vi "ReadJSONFromSerialPort.vi"() -> ()   [LabVIEW 2022 SP3]
uses:
  <vilib>/Analysis/coordinate.llb/Angle Range (Degree).ctl
  <vilib>/Analysis/coordinate.llb/Angle Units.ctl
  <vilib>/Analysis/coordinate.llb/Wrap Angle (scalar).vi
  <vilib>/Instr/_visa.llb/VISA Configure Serial Port (Instr).vi
  <vilib>/addons/control/pid/pid.llb/PID Advanced (DBL).vi
  <vilib>/addons/control/pid/NI_PID_pid.lvlib
  <vilib>/Analysis/NI_AAL_Angle.lvlib
panel:
  in  "auto? (T)":bool=TRUE
  in  "manual output":dbl format="%.2f"
  out "Arduino meas speed RPM":dbl(graph)
  out "LabviewRPM":dbl(graph)
  out "rpm":dbl
  out "angle":dbl(knob) scale=0.0..360.0
  out "force":dbl(graph)
  out "Speed Indicator":dbl=20.0
  in  "Tf [s]":dbl=5.0 caption="Filter time-constant, Tf [s]" min=0.0
  out "PID out":dbl(graph)
  in  "PID gains":T1={"proportional gain (Kc)"=1.0, "integral time (Ti, min)"=0.01, "derivative time (Td, min)"=0.0} {"derivative time (Td, min)" format="%.3f"; "integral time (Ti, min)" format="%.3f"; "proportional gain (Kc)" format="%.3f"}
  in  "setpoint":dbl format="%.2f"
  out "error out 3":errorcluster
  out "measured loop time":dbl
  out "Json out":string
  out "speed chart":T2(graph)
  out "angleChart":dbl(graph)
  in  "stop":bool
  out "angle 2":dbl
  out "error out":errorcluster
  out "Json in":string
  in  "baud rate (115200)":u32=250000
  in  "VISA resource name 2":refnum<visa-resource-name>="COM3"
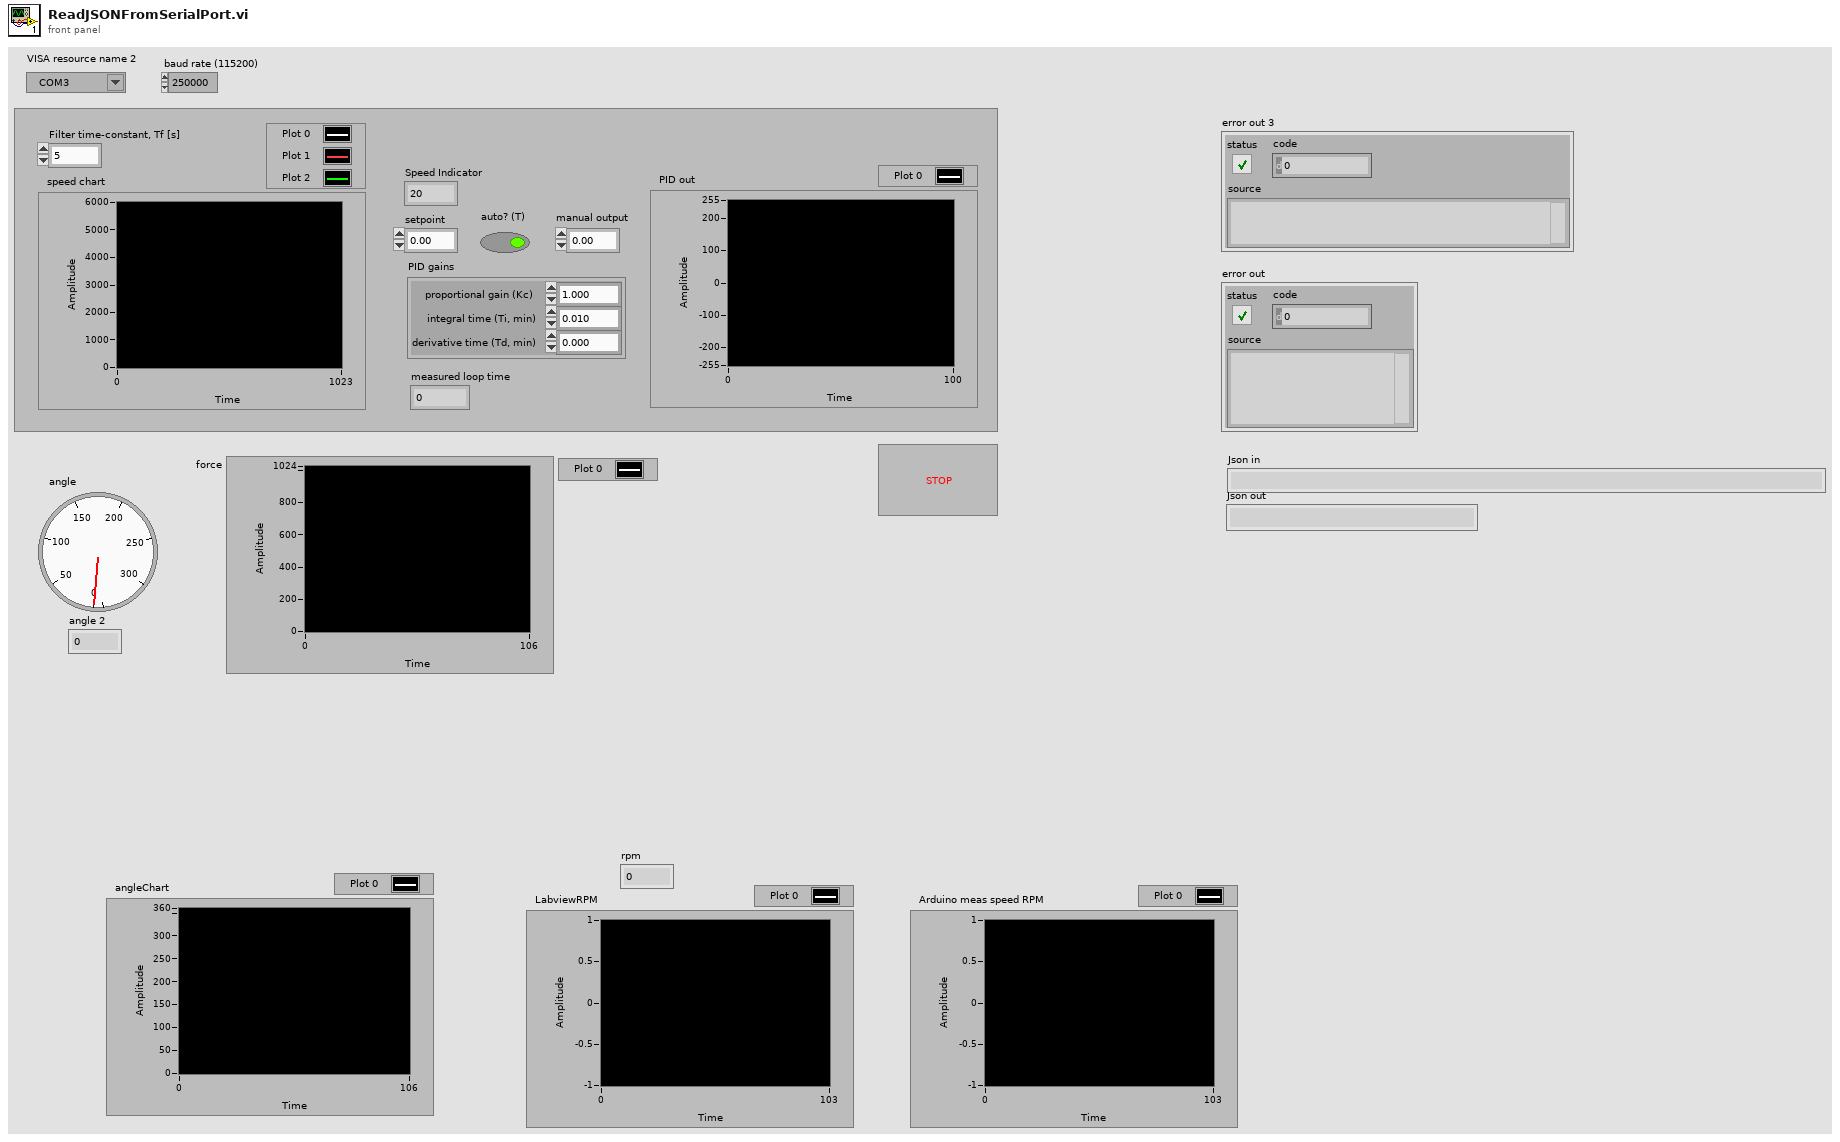
[diagram p1: front panel]
types:
  T1 = cluster{"proportional gain (Kc)":dbl, "integral time (Ti, min)":dbl, "derivative time (Td, min)":dbl}
  T2 = cluster{"setpoint":dbl, "Filter_output":dbl, "speed":dbl}
  T3 = typedef "NI_AAL_Angle.lvlib/Angle Units.ctl" = i32
  T4 = typedef "NI_AAL_Angle.lvlib/Angle Range (Degree).ctl" = u16
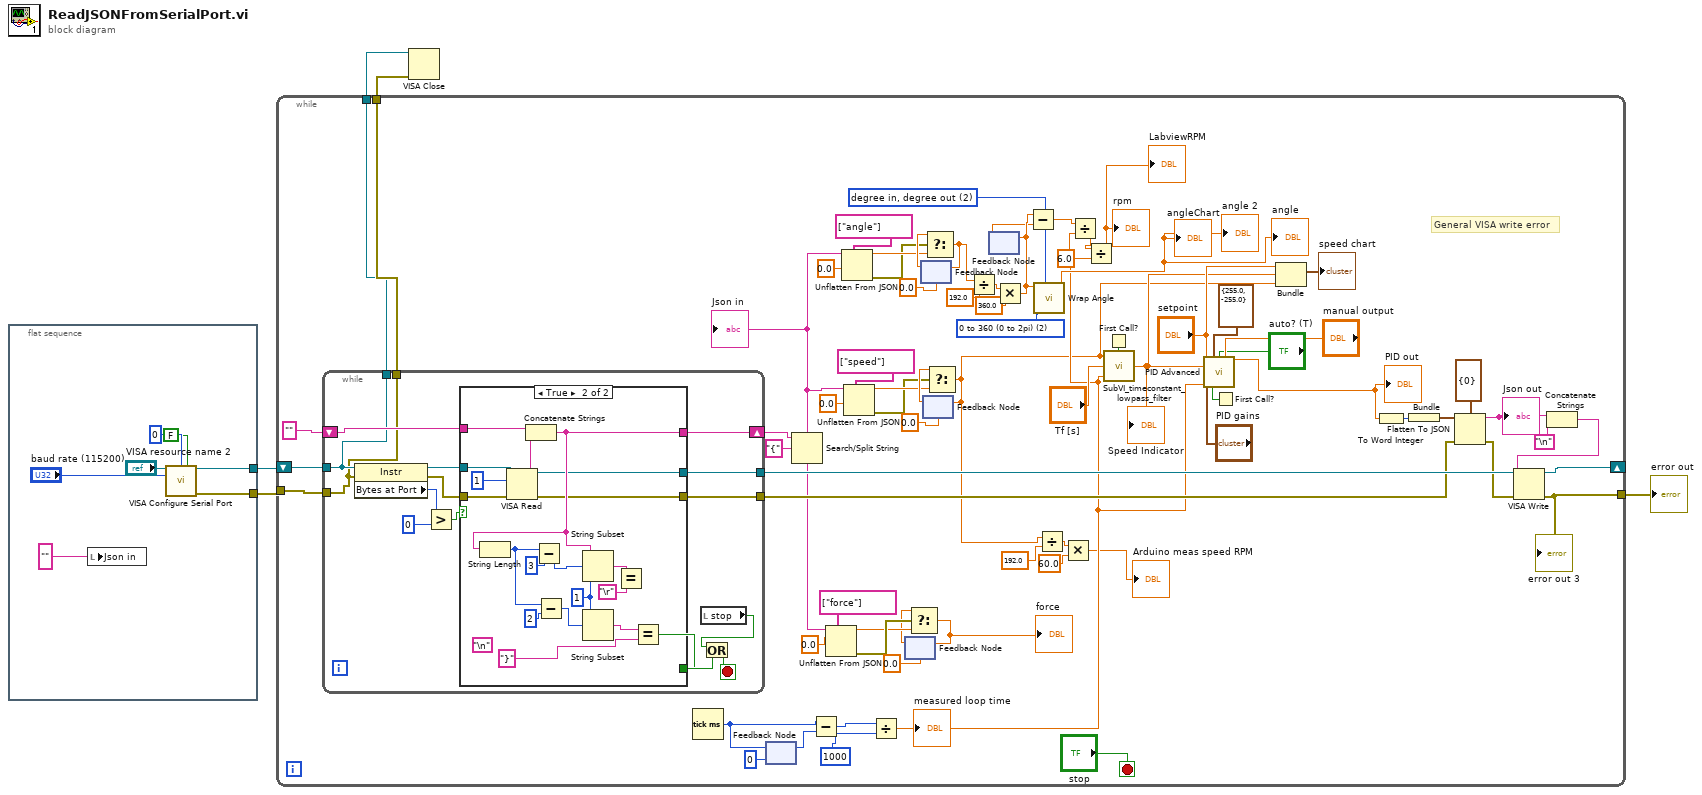
[diagram p0: block diagram]
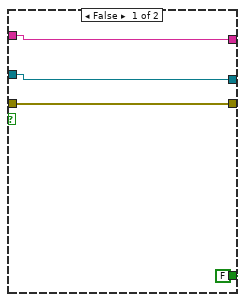
[diagram p2: hidden frame]
diagram:
  n1 = flat-sequence {
    tunnel: [w10] -> w1
    tunnel: [w9] -> w5
    frame #0 {
      n2 = local write "Json in"("" ("data string")) -> ()
      n3 = call-poly "VISA Configure Serial Port"("VISA resource name"="VISA resource name 2", "termination char\n(0xA = '\\n' = LF)"=u8 0 ("termination char\n(0xA = '\\n' = LF)"), "Enable Termination\nChar (T)"=FALSE ("Enable Termination\nChar (T)"), "baud rate (9600)"="baud rate (115200)") -> ("VISA resource name out"=w10:refnum<visa-resource-name>, "error out"=w9:errorcluster)  [unwired: 10 in]
    }
  }
  n4 = while {
    tunnel: w5 -> [w86]
    tunnel: [w84] -> w4
    tunnel: [w83] -> w3
    tunnel: [w71] -> w2
    shift-right: [w67] -> _
    shift-left: w1 -> [w66]
    stop <- "stop" stop-if-true
    w32 = T3 2 items=["radian in, radian out", "radian in, degree out", "degree in, degree out", "degree in, radian out"] ("angle units")
    w33 = T4 2 items=["none", "-180 to 180 (-pi to pi)", "0 to 360 (0 to 2pi)"] ("angle range")
    # "General VISA write error"
    n5 = while {
      tunnel: w66 -> [w93]
      tunnel: w86 -> [w92]
      shift-right: [w95] -> w54
      shift-left: "" -> [w94]
      tunnel: [w93] -> w83
      tunnel: [w92] -> w84
      tunnel: [w91] -> w47
      tunnel: [w87] -> w72
      stop <- w89 stop-if-true
      n6 = property class="Instr"(reference=w93, error in=w92) -> (reference out=w99:refnum<visa-resource-name>, error out=w100:errorcluster, "Bytes at Port"=w98:u32)
      n7 = Greater?(x=w98, y=u32 0) -> (0:w96:bool)
      n8 = case shown="True" w96 {
        tunnel: w100 -> [w102 w123]
        tunnel: w99 -> [w101 w122]
        tunnel: [w104 w112] -> w95
        tunnel: w94 -> [w104 w119]
        tunnel: [FALSE w106] -> w90
        tunnel: [w102 w108] -> w91
        tunnel: [w101 w105] -> w87
        frame False {
        }
        frame True {
          (unwired) "\n"
          w114 = 1 ("length (rest)")
          n9 = VISA Read(VISA resource name=w122, byte count=u32 1, error in (no error)=w123) -> (VISA resource name out=w105:refnum<visa-resource-name>, read buffer=w120:string, error out=w108:errorcluster)  [unwired: 1 out]
          n10 = Concatenate Strings "Concatenate Strings"(w119, w120) -> (w112:string)
          n11 = String Length(string=w112) -> (length=w117:i32)
          n12 = Subtract(x=w117, y=3) -> (x-y=w115:i32)
          n13 = Subtract(x=w117, y=2) -> (x-y=w113:i32)
          n14 = String Subset(string=w112, offset (0)=w115, length (rest)=w114) -> (substring=w111:string)
          n15 = String Subset(string=w112, offset (0)=w113, length (rest)=w114) -> (substring=w109:string)
          n16 = Equal?(x=w111, y="\r") -> ()  [unwired: 1 out]
          n17 = Equal?(x=w109, y="}") -> (x = y?=w106:bool)
        }
      }
      n18 = local read "stop"() -> (w88:bool)
      n19 = Or(x=w88, y=w90) -> (x .or. y?=w89:bool)
    }
    n20 = Tick Count (ms)() -> (millisecond timer value=w76:u32)
    n21 = feedback-in #1(w76) -> ()
    n22 = feedback #1(u32 0 ("millisecond timer value")) -> (w77:u32)
    n23 = Search/Split String(string=w54, search string/char (-)="{") -> (match + rest of string=w34:string)  [unwired: 1 in, 2 out]
    "Json in" <- w34
    n24 = Subtract(x=w76, y=w77) -> (x-y=w75:u32)
    n25 = Unflatten From JSON(path=string[] ["force"], JSON string=w34, type and defaults=0.0 ("speed")) -> (value=w51:dbl, error out=w52:errorcluster)  [unwired: 4 in]
    n26 = Unflatten From JSON(path=string[] ["angle"], JSON string=w34, type and defaults=0.0 ("speed")) -> (value=w45:dbl, error out=w44:errorcluster)  [unwired: 4 in]
    n27 = Unflatten From JSON(path=string[] ["speed"], JSON string=w34, type and defaults=0.0 ("speed")) -> (value=w39:dbl, error out=w38:errorcluster)  [unwired: 4 in]
    n28 = Divide(x=w75, y=u32 1000) -> (x/y=w23:dbl)
    "measured loop time" <- w23
    n29 = feedback #2(0.0 ("speed")) -> (w50:dbl)
    n30 = Select(t=w50, s=w52, f=w51) -> (s? t:f=w49:dbl)
    "force" <- w49
    n31 = feedback-in #2(w49) -> ()
    n32 = feedback #3(0.0 ("speed")) -> (w46:dbl)
    n33 = feedback #4(0.0 ("speed")) -> (w40:dbl)
    n34 = Select(t=w46, s=w44, f=w45) -> (s? t:f=w31:dbl)
    n35 = feedback-in #3(w31) -> ()
    n36 = Select(t=w40, s=w38, f=w39) -> (s? t:f=w17:dbl)
    n37 = feedback-in #4(w17) -> ()
    n38 = Divide(x=w31, y=192.0) -> (x/y=w29:dbl)
    n39 = feedback #5() -> (w25:dbl)  [unwired: 1 in]
    n40 = Multiply(x=w29, y=360.0) -> (x*y=w26:dbl)
    n41 = feedback-in #5(w26) -> ()
    n42 = Subtract(x=w26, y=w25) -> (x-y=w24:dbl)
    n43 = call-poly <vilib>:"Wrap Angle.vi"("angle units"=w32, "angle range"=w33, "angle in"=w26) -> ("angle out"=→"angle 2" →"angleChart" →"angle":dbl)  [unwired: 7 in, 1 out]
    n44 = Divide(x=w17, y=192.0) -> (x/y=w16:dbl)
    n45 = Multiply(x=w16, y=60.0) -> (x*y=→"Arduino meas speed RPM":dbl)
    n46 = Divide(x=w24, y=w23) -> (x/y=w22:dbl)
    n47 = Divide(x=w22, y=6.0) -> (x/y=→"rpm" →"LabviewRPM":dbl)
    n48 = First Call?() -> (First Call?: T/F=w61:bool)
    n49 = call "SubVI_timeconstant_lowpass_filter.vi"("Init/reset"=w61, "Ts [s]"=w23, "Tf [s]"="Tf [s]", "Filter_input"=w17) -> ("Filter_output"=w58:dbl)
    "Speed Indicator" <- w58
    n50 = First Call?() -> (First Call?: T/F=w60:bool)
    n51 = call-poly <vilib>:"PID Advanced.vi"("setpoint"="setpoint", "output range"=cluster{"output high":dbl, "output low":dbl} {"output high"=255.0, "output low"=-255.0}, "auto? (T)"="auto? (T)", "manual control"="manual output", "process variable"=w58, "PID gains"="PID gains", "dt (s)"=w23, "reinitialize? (F)"=w60) -> ("output"=w63:dbl)  [unwired: 6 in, 1 out]
    "PID out" <- w63
    n52 = Bundle("setpoint"="setpoint", "Filter_output"=w58, "speed"=w17) -> (→"speed chart":T2)  [unwired: 1 in]
    n53 = To Word Integer(number=w63) -> (16bit integer=w73:i16)
    n54 = Bundle(cluster=cluster{"mv":i32} {"mv"=0}, "mv"=w73) -> (w80:cluster{"mv":i32})
    n55 = Flatten To JSON(anything=w80, error in (no error)=w47) -> (JSON string=w69:string, 11:w68:errorcluster)  [unwired: 1 in]
    "Json out" <- w69
    n56 = Concatenate Strings(w69, "\n") -> (w64:string)
    n57 = VISA Write(VISA resource name=w72, write buffer=w64, error in (no error)=w68) -> (VISA resource name out=w67:refnum<visa-resource-name>, error out=w71:errorcluster)  [unwired: 1 out]
    "error out 3" <- w71
  }
  "error out" <- w2
  n58 = VISA Close(VISA resource name=w3, error in (no error)=w4) -> ()  [unwired: 1 out]
